vi "getVales.vi"(8 "error in (no error)":errorcluster, 10 "phase":T1, 11 "reference in":refnum<class "subject.lvclass">) -> (0 "error out":errorcluster, 3 "reference out":refnum<class "subject.lvclass">)   [LabVIEW 2015, in "subject.lvclass"]
uses:
  subject.lvclass
  phase.ctl
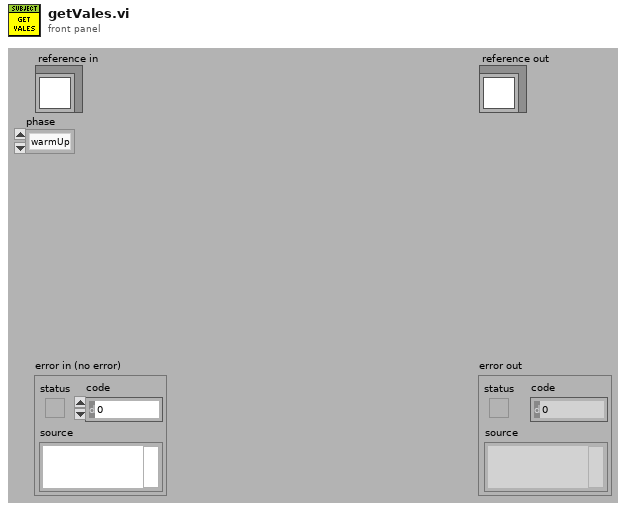
[diagram p1: front panel]
types:
  T1 = typedef "subject.lvclass/phase.ctl" = enum16{"warmUp", "userSelection", "Exercise"}
  T2 = cluster{"peaksAmplitude":dbl[], "iPeaksLocation":dbl[], "valesAmplitude":dbl[], "iValesLocation":dbl[], "threshold":dbl, "warmup_offset":i32, "exer_offset":i32, "#_peaks":i32}
  T3 = typedef "subject.lvclass/ObjectAttributesRef.ctl" = refnum<data-value>
  T4 = typedef "subject.lvclass/ObjectAttributes.ctl" = cluster{"MyAttribute":dbl, "data":cluster{"Ve_warm":dbl[], "time_warm":dbl[], "name":string, "phase":dbl[], "VCO2":dbl[], "VO2":dbl[], "PetCO2":dbl[], "RQ":dbl[], "HR":dbl[], "Ve_warm_inter":dbl[], "time_warm_inter":dbl[], "Ve_exer":dbl[], "time_exer":dbl[], "Ve_exer_inter":dbl[], "time_exer_inter":dbl[], "Ve":dbl[], "time":dbl[], "Ve_exer_inter_filtered":dbl[], "Ve_warm_inter_filtered":dbl[]}, "results_5l":cluster{"EOV":bool, "osci_amplitude":dbl[], "osci_width":dbl[], "peak_location":dbl[], "threshold":dbl, "width":i32}, "results_15percent":cluster{"EOV":bool, "osci_amplitude":dbl[], "osci_width":dbl[], "peak_location":dbl[], "threshold":dbl, "width":i32}, "supportData":cluster{"peaksAmplitude":dbl[], "iPeaksLocation":dbl[], "valesAmplitude":dbl[], "iValesLocation":dbl[], "threshold":dbl, "meanAmpl_warm":i32, "#_peaks":i32, "width":i32}, "results_user_selection":cluster{"EOV":bool, "osci_amplitude":dbl[], "osci_width":dbl[], "peak_location":dbl[], "threshold":dbl, "width":i32}, "results_warm_up":cluster{"EOV":bool, "osci_amplitude":dbl[], "osci_width":dbl[], "peak_location":dbl[], "threshold":dbl, "width":i32}}
  T5 = cluster{"Ve_warm":dbl[], "time_warm":dbl[], "name":string, "phase":dbl[], "VCO2":dbl[], "VO2":dbl[], "PetCO2":dbl[], "RQ":dbl[], "HR":dbl[], "Ve_warm_inter":dbl[], "time_warm_inter":dbl[], "Ve_exer":dbl[], "time_exer":dbl[], "Ve_exer_inter":dbl[], "time_exer_inter":dbl[], "Ve":dbl[], "time":dbl[], "Ve_exer_inter_filtered":dbl[], "Ve_warm_inter_filtered":dbl[]}
  T6 = cluster{"peaksAmplitude":dbl[], "iPeaksLocation":dbl[], "valesAmplitude":dbl[], "iValesLocation":dbl[], "threshold":dbl, "meanAmpl_warm":i32, "#_peaks":i32, "width":i32}
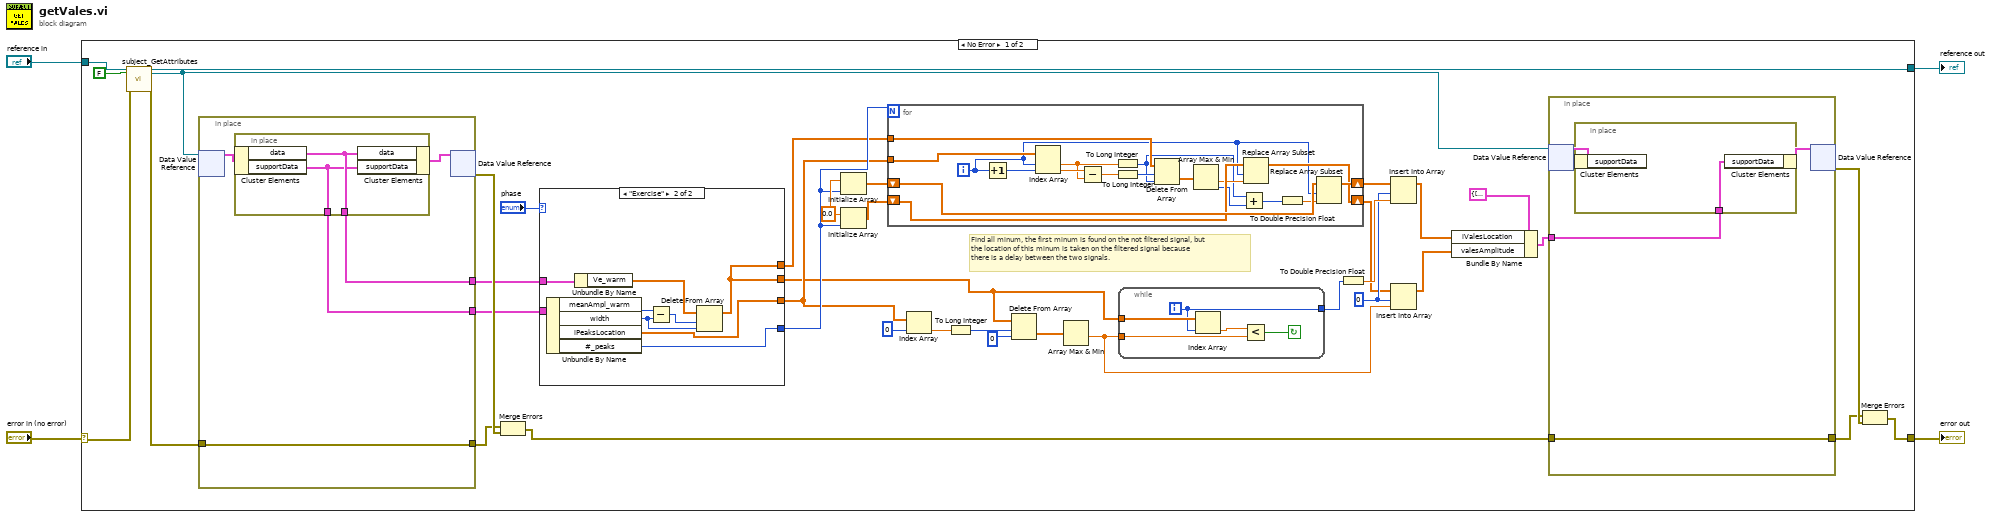
[diagram p0: block diagram]
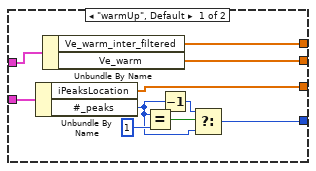
[diagram p2: hidden frame]
diagram:
  n1 = case shown="No Error" "error in (no error)" {
    selector: "error in (no error)" -> [w37 w97]
    tunnel: [w9 w97] -> w3
    tunnel: [w35 w96] -> w1
    tunnel: "reference in" -> [w39 w96]
    frame No Error {
      w28 = 0 ("index")
      w23 = 0.0 ("element")
      # "Find all minum, the first minum is found on the not filtered signal, but the location of this minum is taken on the filtered signal because there is a delay between the two signals."
      n2 = call "subject_GetAttributes.vi"("reference in"=w39, "return data? (T)"=FALSE, "error in (no error)"=w37) -> ("reference out"=w35:refnum<class "subject.lvclass">, "attributes ref"=w16:T3, "error out"=w36:errorcluster)  [unwired: 13 in, 1 out]
      n3 = in-place {
        in-place-border: w36 -> [w91]
        in-place-border: [w91] -> w40
        in-place-border: [w90] -> w34
        in-place-border: [w89] -> w18
        n4 = in-place-dvr #1(w16) -> (w92:T4)  [unwired: 1 out]
        n5 = in-place {
          in-place-border: [w95] -> w90
          in-place-border: [w94] -> w89
          n6 = in-place-cluster #2(w92) -> ("data"=w95:T5, "supportData"=w94:T6)
          n7 = in-place-cluster #2("data"=w95, "supportData"=w94) -> (w93:T4)
        }
        n8 = in-place-dvr #1(w93) -> (w41:errorcluster)  [unwired: 1 out]
      }
      n9 = Merge Errors(w40, w41) -> (w17:errorcluster)
      n10 = case shown="\"Exercise\"" "phase" {
        tunnel: w34 -> [w79 w88]
        tunnel: w18 -> [w78 w87]
        tunnel: [w73 w81] -> w8
        tunnel: [w72 w82] -> w7
        tunnel: [w71 w80] -> w6
        tunnel: [w70 w80] -> w5
        frame "warmUp", Default {
          n11 = Unbundle By Name(w78) -> ("iPeaksLocation"=w72:dbl[], "#_peaks"=w74:i32)
          n12 = Unbundle By Name(w79) -> ("Ve_warm_inter_filtered"=w71:dbl[], "Ve_warm"=w70:dbl[])
          n13 = Equal?(x=w74, y=1) -> (x = y?=w76:bool)
          n14 = Decrement(x=w74) -> (x-1=w75:i32)
          n15 = Select(t=w75, s=w76, f=w74) -> (s? t:f=w73:i32)
        }
        frame "Exercise" {
          n16 = Unbundle By Name(w87) -> ("meanAmpl_warm"=w85:i32, "width"=w83:i32, "iPeaksLocation"=w82:dbl[], "#_peaks"=w81:i32)
          n17 = Unbundle By Name(w88) -> ("Ve_warm"=w86:dbl[])
          n18 = Subtract(x=w85, y=w83) -> (x-y=w84:i32)
          n19 = Delete From Array(array=w86, length=w84, index=w83) -> (array with subset deleted=w80:dbl[])  [unwired: 1 out]
        }
      }
      n20 = Initialize Array(w23, w8) -> (w25:dbl[])
      n21 = Initialize Array(w23, w8) -> (w24:dbl[])
      n22 = for {
        N: w8 -> [_]
        tunnel: w6 -> [w69]
        tunnel: w7 -> [w68]
        shift-right: [w60] -> w27
        shift-left: w25 -> [w61]
        shift-right: [w58] -> w26
        shift-left: w24 -> [w59]
        i -> [w57]
        n23 = Increment(x=w57) -> (x+1=w67:i32)
        n24 = Index Array(array=w68, index #1=w57, index #2=w67) -> (element #1=w65:dbl, element #2=w66:dbl)
        n25 = Subtract(x=w66, y=w65) -> (x-y=w64:dbl)
        n26 = To Long Integer(number=w65) -> (32bit integer=w52:i32)
        n27 = To Long Integer(number=w64) -> (32bit integer=w63:i32)
        n28 = Delete From Array(array=w69, length=w63, index=w52) -> (deleted portion=w62:dbl[])  [unwired: 1 out]
        n29 = Array Max & Min(array=w62) -> (min value=w56:dbl, min index (indices)=w55:i32)  [unwired: 2 out]
        n30 = Add(x=w52, y=w55) -> (x+y=w53:i32)
        n31 = Replace Array Subset(array=w59, new element=w56, index=w57) -> (w58:dbl[])
        n32 = To Double Precision Float(number=w53) -> (double precision float=w54:dbl)
        n33 = Replace Array Subset(array=w61, new element=w54, index=w57) -> (w60:dbl[])
      }
      n34 = Index Array(array=w7, index=0) -> (element=w20:dbl)
      n35 = To Long Integer(number=w20) -> (32bit integer=w30:i32)
      n36 = Delete From Array(array=w5, length=w30, index=0) -> (deleted portion=w22:dbl[])  [unwired: 1 out]
      n37 = Array Max & Min(array=w22) -> (min value=w29:dbl)  [unwired: 3 out]
      n38 = while {
        tunnel: w29 -> [w49]
        tunnel: w5 -> [w51]
        tunnel: [w47] -> w31
        i -> [w47]
        stop <- w48 continue-if-true
        n39 = Index Array(array=w51, index=w47) -> (element=w50:dbl)
        n40 = Less?(x=w50, y=w49) -> (x < y?=w48:bool)
      }
      n41 = To Double Precision Float(number=w31) -> (double precision float=w32:dbl)
      n42 = Insert Into Array(array=w27, index=w28, new element=w32) -> (w14:dbl[])
      n43 = Insert Into Array(array=w26, index=w28, new element=w29) -> (w12:dbl[])
      n44 = Bundle By Name(cluster=T2 {"peaksAmplitude"=[], "iPeaksLocation"=[], "valesAmplitude"=[], "iValesLocation"=[], "threshold"=0.0, "warmup_offset"=0, "exer_offset"=0, "#_peaks"=0} ("supportData"), "iValesLocation"=w14, "valesAmplitude"=w12) -> (w13:T2)
      n45 = in-place {
        in-place-border: w17 -> [w43]
        in-place-border: [w43] -> w10
        in-place-border: w13 -> [w42]
        n46 = in-place-dvr #3(w16) -> (w44:T4)  [unwired: 1 out]
        n47 = in-place {
          in-place-border: w42 -> [w46]
          n48 = in-place-cluster #4(w44) -> ()  [unwired: 1 out]
          n49 = in-place-cluster #4("supportData"=w46) -> (w45:T4)
        }
        n50 = in-place-dvr #3(w45) -> (w11:errorcluster)  [unwired: 1 out]
      }
      n51 = Merge Errors(w10, w11) -> (w9:errorcluster)
    }
    frame Error {
    }
  }
  "error out" <- w3
  "reference out" <- w1
